vi "Array_2_delimited_string.vi"(9 "delimiter (Tab)":string, 11 "Array of Strings":string[](array[string])) -> (2 "delimited string":string)   [LabVIEW 2011]
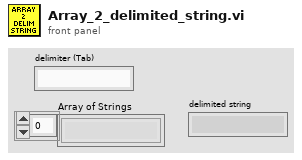
[diagram p1: front panel]
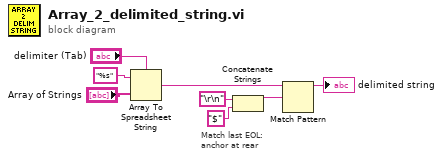
[diagram p0: block diagram]
diagram:
  # "Match last EOL:\nanchor at rear"
  n1 = Array To Spreadsheet String(delimiter (Tab)="delimiter (Tab)", array="Array of Strings", 3:"%s" ("format string")) -> (spreadsheet string=w2:string)
  n2 = Concatenate Strings("\r\n", "$" ("Substring")) -> (w3:string)
  n3 = Match Pattern(string=w2, regular expression=w3) -> (before substring=→"delimited string":string)  [unwired: 1 in, 3 out]
